vi "Controller.vi"(8 "error in":errorcluster) -> ()   [LabVIEW 2014, in "Elevator System.lvlib"]
uses:
  Elevator System.lvlib
  Typedef/MessageType.ctl
  Typedef/Commands.ctl
  Typedef/GripperNotifierType.ctl
  Typedef/ControllerStateData.ctl
  Typedef/ControllerStates.ctl
  Typedef/StackMessage.ctl
  Typedef/StackCommandType.ctl
  Typedef/TeirNumber.ctl
  Sensors Global.vi
panel:
  in  "Loops":i32=7
  in  "Tolerance 2":dbl=0.015 format="%#_13g"
  in  "Tolerance":dbl=0.04 format="%#_13g"
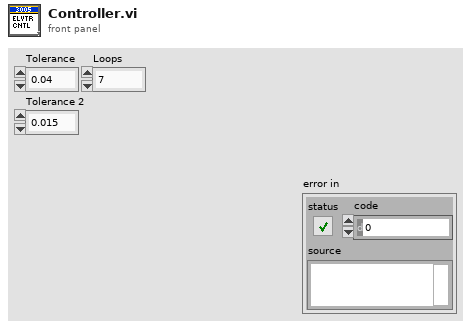
[diagram p1: front panel]
types:
  T1 = typedef "Elevator System.lvlib/ControllerStates.ctl" = enum16{"Init", "Set Elevator SP", "Set Gripper SP", "Wait For Elevator", "Wait For Gripper", "Wait For Elevator Fast", "Wait For Gripper Fast", "Disabled"}
  T2 = typedef "Elevator System.lvlib/ControllerStateData.ctl" = cluster{"State":T1, "Data":dbl[]}
  T3 = cluster{"Elevator":refnum<notifier>, "Gripper":refnum<notifier>}
  T4 = typedef "Elevator System.lvlib/Commands.ctl" = enum16{"Home", "Stack", "Pickup", "Score", "Cycle", "Stop", "Manual Open", "Manual Close", "Manual Up", "Manual Down", "Gripper RC", "Gripper Cycle", "Wait On Gripper", "Wait On Elevator"}
  T5 = typedef "Elevator System.lvlib/MessageType.ctl" = cluster{"Name":T4, "Data":variant}
  T6 = typedef "Elevator System.lvlib/StackMessage.ctl" = cluster{"Type":T7, "Teir":T8}
  T7 = typedef "Elevator System.lvlib/StackCommandType.ctl" = enum16{"Normal", "RC", "Step"}
  T8 = typedef "Elevator System.lvlib/TeirNumber.ctl" = enum16{"T1", "T2", "T3", "T4", "T5", "T6"}
  T9 = typedef "Elevator System.lvlib/GripperNotifierType.ctl" = cluster{"SP Left":dbl, "SP Right":dbl}
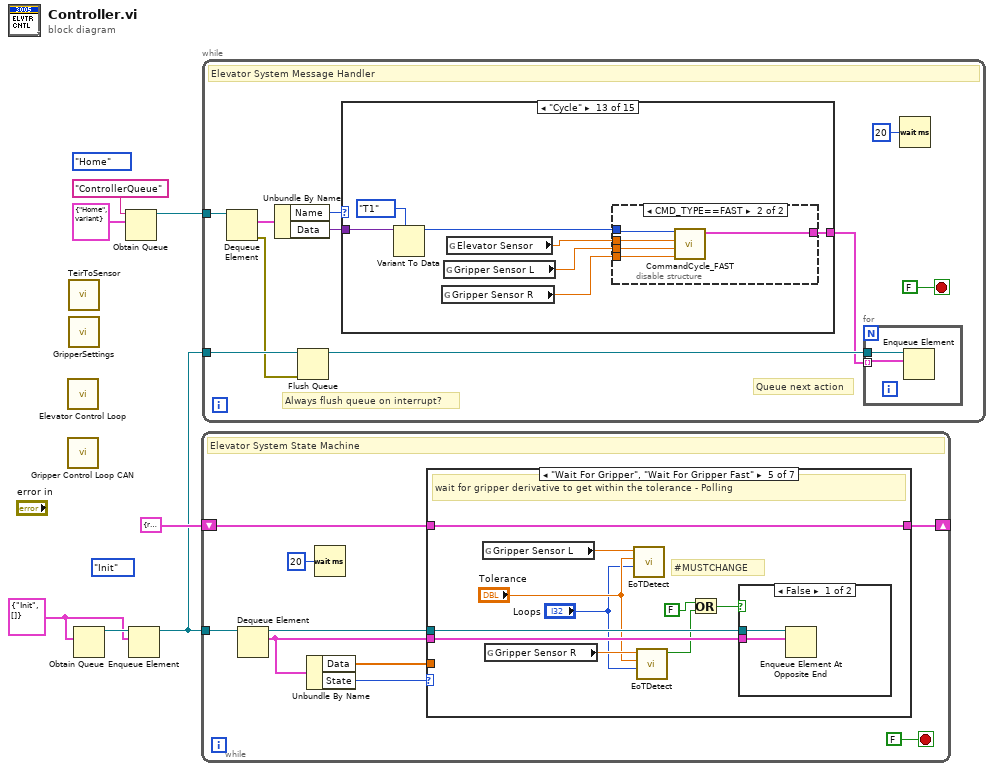
[diagram p0: block diagram]
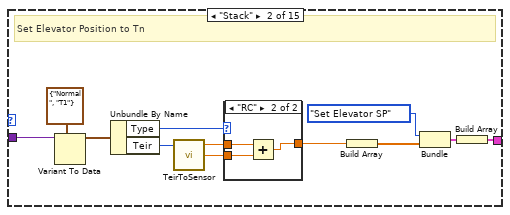
[diagram p3: hidden frame]
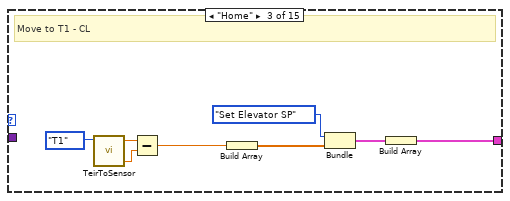
[diagram p5: hidden frame]
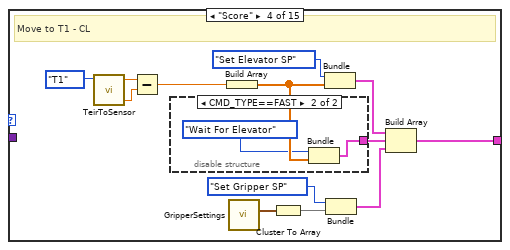
[diagram p6: hidden frame]
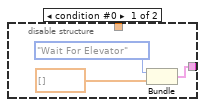
[diagram p7: hidden frame]
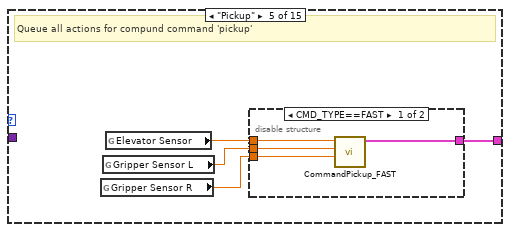
[diagram p8: hidden frame]
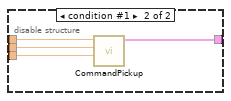
[diagram p9: hidden frame]
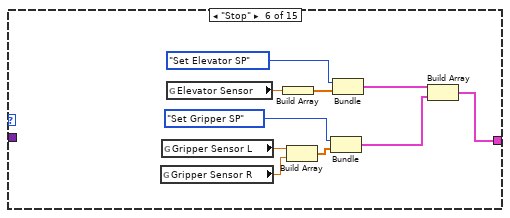
[diagram p10: hidden frame]
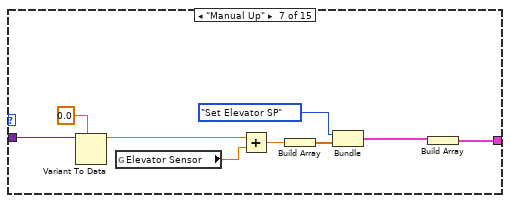
[diagram p11: hidden frame]
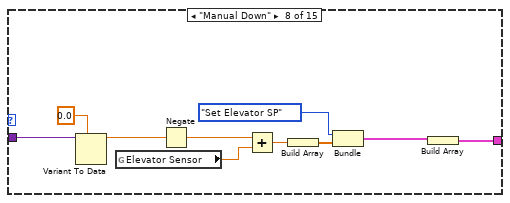
[diagram p12: hidden frame]
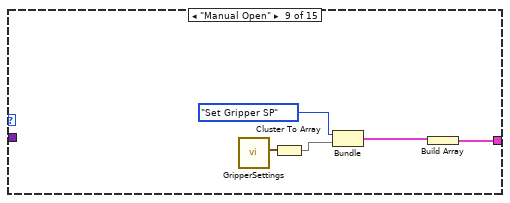
[diagram p13: hidden frame]
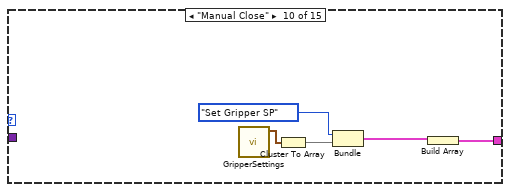
[diagram p14: hidden frame]
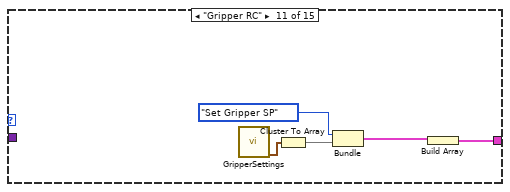
[diagram p15: hidden frame]
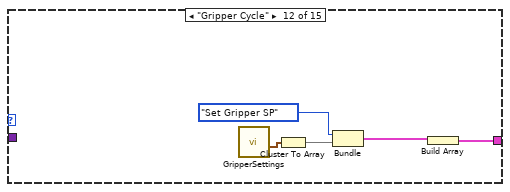
[diagram p16: hidden frame]
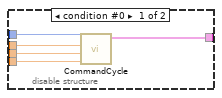
[diagram p17: hidden frame]
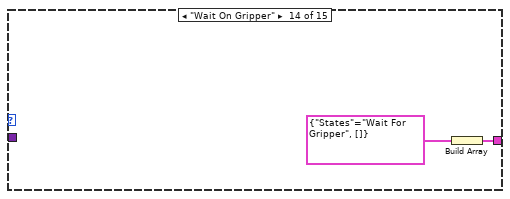
[diagram p18: hidden frame]
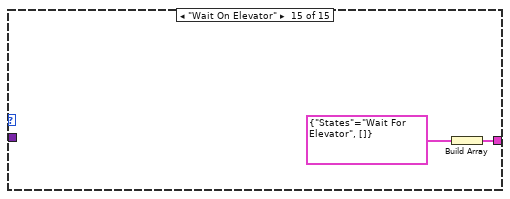
[diagram p19: hidden frame]
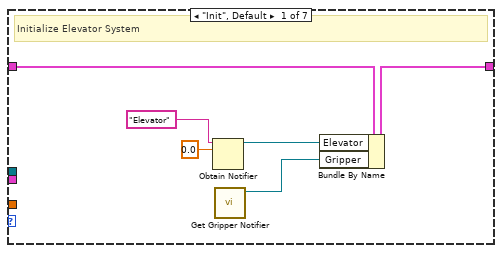
[diagram p20: hidden frame]
diagram:
  (unwired) ControllerStates."Init" ("State")
  w1 = T2 {"State"=enum."Init", "Data"=[]}
  (unwired) Commands."Home" ("Name")
  n1 = call "Elevator Control Loop.vi"() -> ()  [unwired: 12 in]
  n2 = call "Gripper Control Loop CAN.vi"() -> ()  [unwired: 12 in]
  n3 = call "TeirToSensor.vi"() -> ()  [unwired: 4 in, 5 out]
  n4 = call "GripperSettings.vi"() -> ()  [unwired: 5 in, 5 out]
  n5 = Obtain Queue(element data type=w1) -> (queue out=w4:refnum<queue>)  [unwired: 4 in, 2 out]
  n6 = Obtain Queue(name (unnamed)="ControllerQueue", element data type=T5 {"Name"=enum."Home", "Data"=variant} ("Message")) -> (queue out=w5:refnum<queue>)  [unwired: 3 in, 2 out]
  n7 = Enqueue Element(queue=w4, element=w1) -> (queue out=w2:refnum<queue>)  [unwired: 2 in, 2 out]
  n8 = while {
    tunnel: w2 -> [w14]
    shift-right: [w11] -> _
    shift-left: T3 {"Elevator"=refnum, "Gripper"=refnum} -> [w12]
    stop <- FALSE stop-if-true
    # "Elevator System State Machine"
    n9 = Dequeue Element(queue=w14) -> (queue out=w13:refnum<queue>, element=w10:T2)  [unwired: 2 in, 2 out]
    n10 = Unbundle By Name(w10) -> ("Data"=w8:dbl[], "State"=w9:T1)
    n11 = Wait (ms)(milliseconds to wait=u32 20) -> ()  [unwired: 1 out]
    n12 = case shown="\"Wait For Gripper\", \"Wait For Gripper Fast\"" w9 {
      tunnel: w13 -> [_ _ _ w36 w50 w65 w86]
      tunnel: w12 -> [w20 w29 w33 w39 w52 w66 w87]
      tunnel: [w19 w29 w33 w39 w52 w66 w87] -> w11
      tunnel: w10 -> [_ _ _ w35 w49 w64 w85]
      tunnel: w8 -> [_ w24 w30 _ _ w63 w77]
      frame "Init", Default {
        # "Initialize Elevator System"
        n13 = Obtain Notifier(name (unnamed)="Elevator", notification data type=0.0) -> (notifier out=w21:refnum<notifier>)  [unwired: 2 in, 2 out]
        n14 = call "Get Gripper Notifier.vi"() -> ("Notifier out"=w17:refnum<notifier>)  [unwired: 11 in]
        n15 = Bundle By Name(cluster=w20, "Elevator"=w21, "Gripper"=w17) -> (w19:T3)
      }
      frame "Set Elevator SP" {
        # "Set the Elevator PID Setpoint"
        n16 = Index Array(array=w24) -> (element=w23:dbl)  [unwired: 1 in]
        n17 = call "TeirToSensor.vi"() -> ("Max"=w26:dbl, "Min"=w25:dbl)  [unwired: 4 in, 3 out]
        n18 = Unbundle By Name(w29) -> ("Elevator"=w28:refnum<notifier>)
        n19 = In Range and Coerce(upper limit=w26, x=w23, lower limit=w25) -> (coerced(x)=w27:dbl)  [unwired: 1 out]
        n20 = Send Notification(notification=w27, notifier=w28) -> ()  [unwired: 1 in, 2 out]
      }
      frame "Set Gripper SP" {
        # "Set the Gripper PID Setpoint"
        n21 = Array To Cluster(array=w30) -> (cluster=w31:cluster{"Data[0]":dbl, "Data[1]":dbl})
        n22 = Unbundle By Name(w33) -> ("Gripper"=w32:refnum<notifier>)
        n23 = Send Notification(notification=w31, notifier=w32) -> ()  [unwired: 1 in, 2 out]
      }
      frame "Wait For Elevator" {
        # "wait for elevator derivative to get within the tolerance - Polling"
        n24 = global read "Sensors Global.vi" "Elevator Sensor"() -> (w38:dbl)
        n25 = call "EoTDetect.vi"("Tolerance"="Tolerance 2", "Sensor"=w38) -> ("EoT? (F)"=w34:bool)  [unwired: 9 in]
        n26 = case shown="False" w34 {
          tunnel: w36 -> [w41 _]
          tunnel: w35 -> [w40 _]
          frame False {
            n27 = Enqueue Element At Opposite End(queue=w41, element=w40) -> ()  [unwired: 2 in, 3 out]
          }
          frame True {
            n28 = call "GetElevatorStatus.vi"("Action"=enum16{"Get", "Set", "Clear"}."Set") -> ()  [unwired: 10 in, 1 out]
          }
        }
      }
      frame "Wait For Gripper", "Wait For Gripper Fast" {
        # "#MUSTCHANGE"
        # "wait for gripper derivative to get within the tolerance - Polling"
        n29 = global read "Sensors Global.vi" "Gripper Sensor L"() -> (w51:dbl)
        n30 = global read "Sensors Global.vi" "Gripper Sensor R"() -> (w48:dbl)
        n31 = call "EoTDetect.vi"("Loops"="Loops", "Tolerance"="Tolerance", "Sensor"=w51) -> ()  [unwired: 8 in, 1 out]
        n32 = call "EoTDetect.vi"("Loops"="Loops", "Tolerance"="Tolerance", "Sensor"=w48) -> ("EoT? (F)"=w44:bool)  [unwired: 8 in]
        n33 = Or(x=FALSE ("y"), y=w44) -> (x .or. y?=w47:bool)
        n34 = case shown="False" w47 {
          tunnel: w50 -> [w54 _]
          tunnel: w49 -> [w53 _]
          frame False {
            n35 = Enqueue Element At Opposite End(queue=w54, element=w53) -> ()  [unwired: 2 in, 3 out]
          }
          frame True {
            n36 = call "GetGripperStatus.vi"("Action"=enum16{"Get", "Set", "Clear"}."Set") -> ()  [unwired: 10 in, 1 out]
          }
        }
      }
      frame "Wait For Elevator Fast" {
        # "-1 = Going Down\n1 = going up"
        # "Wait for Elevator to get to a position - Polling"
        n37 = call "TeirToSensor.vi"() -> ("Max"=w58:dbl)  [unwired: 4 in, 4 out]
        n38 = global read "Sensors Global.vi" "Elevator Sensor"() -> (w62:dbl)
        n39 = Index Array(array=w63) -> (element #1=w61:dbl, element #2=w56:dbl)  [unwired: 2 in]
        n40 = In Range and Coerce(upper limit=w58, x=w61, lower limit=0.3) -> (coerced(x)=w59:dbl)  [unwired: 1 out]
        n41 = case shown="-1, Default" w56 {
          tunnel: w62 -> [w69 w72]
          tunnel: w59 -> [w68 w71]
          tunnel: [w67 w70] -> w60
          frame 1 {
            n42 = Greater Or Equal?(x=w69, y=w68) -> (x >= y?=w67:bool)
          }
          frame -1, Default {
            n43 = Less Or Equal?(x=w72, y=w71) -> (x <= y?=w70:bool)
          }
        }
        n44 = case shown="False" w60 {
          tunnel: w65 -> [w74 _]
          tunnel: w64 -> [w73 _]
          frame False {
            n45 = Enqueue Element At Opposite End(queue=w74, element=w73) -> ()  [unwired: 2 in, 3 out]
          }
          frame True {
            n46 = call "GetElevatorStatus.vi"("Action"=enum16{"Get", "Set", "Clear"}."Set") -> ()  [unwired: 10 in, 1 out]
          }
        }
      }
      frame "Disabled" {
        # "Wait for Elevator to get to target position - Polling"
        n47 = global read "Sensors Global.vi" "Gripper Sensor L"() -> (w82:dbl)
        n48 = global read "Sensors Global.vi" "Gripper Sensor R"() -> (w81:dbl)
        n49 = Build Array(w82, w81) -> (w80:dbl[])
        n50 = Subtract(x=w80, y=w77) -> (x-y=w84:dbl[])
        n51 = Absolute Value(x=w84) -> (abs(x)=w83:dbl[])
        n52 = call "GripperSettings.vi"() -> ("Detect Tolerance"=w76:dbl)  [unwired: 5 in, 4 out]
        n53 = Less?(x=w83, y=w76) -> (x < y?=w78:bool[])
        n54 = And Array Elements(Boolean array=w78) -> (logical AND=w79:bool)
        n55 = case shown="False" w79 {
          tunnel: w86 -> [w89 _]
          tunnel: w85 -> [w88 _]
          frame False {
            n56 = Enqueue Element At Opposite End(queue=w89, element=w88) -> ()  [unwired: 2 in, 3 out]
          }
          frame True {
            n57 = call "GetElevatorStatus.vi"("Action"=enum16{"Get", "Set", "Clear"}."Set") -> ()  [unwired: 10 in, 1 out]
          }
        }
      }
    }
  }
  n58 = while {
    tunnel: w5 -> [w96]
    tunnel: w2 -> [w97]
    stop <- FALSE stop-if-true
    # "Queue next action"
    # "Always flush queue on interrupt?"
    # "Elevator System Message Handler"
    n59 = Dequeue Element(queue=w96) -> (element=w95:T5, error out=w92:errorcluster)  [unwired: 2 in, 2 out]
    n60 = Unbundle By Name(w95) -> ("Name"=w99:T4, "Data"=w98:variant)
    n61 = Flush Queue(queue=w97, error in (no error)=w92) -> (queue out=w100:refnum<queue>)  [unwired: 2 out]
    n62 = case shown="\"Cycle\"" w99 {
      tunnel: w98 -> [_ w112 _ _ _ _ w169 w179 _ _ _ _ w208 _ _]
      tunnel: [_ w109 w122 w135 w147 w163 w172 w182 w187 w192 w197 w202 w211 w222 w224] -> w94
      frame Default {
      }
      frame "Stack" {
        # "Set Elevator Position to Tn"
        n63 = Variant To Data(type=T6 {"Type"=enum."Normal", "Teir"=enum."T1"}, Variant=w112) -> (data=w107:T6)  [unwired: 1 in, 1 out]
        n64 = Unbundle By Name(w107) -> ("Type"=w102:T7, "Teir"=w106:T8)
        n65 = call "TeirToSensor.vi"("Enum"=w106) -> ("T1"=w105:dbl, "CR"=w104:dbl)  [unwired: 3 in, 3 out]
        n66 = case shown="\"RC\"" w102 {
          tunnel: w105 -> [w113 w116]
          tunnel: w104 -> [_ w115]
          tunnel: [w113 w114] -> w103
          frame "Normal", Default {
          }
          frame "RC" {
            n67 = Add(x=w116, y=w115) -> (x+y=w114:dbl)
          }
        }
        n68 = Build Array(w103) -> (w101:dbl[])
        n69 = Bundle("States"=ControllerStates."Set Elevator SP", w101) -> (w110:cluster{"States":T1, dbl[]})  [unwired: 1 in]
        n70 = Build Array(w110) -> (w109:cluster{"States":T1, dbl[]}[])
      }
      frame "Home" {
        # "Move to T1 - CL"
        n71 = call "TeirToSensor.vi"("Enum"=TeirNumber."T1") -> ("T1"=w120:dbl, "CL"=w119:dbl)  [unwired: 3 in, 3 out]
        n72 = Subtract(x=w120, y=w119) -> (x-y=w118:dbl)
        n73 = Build Array(w118) -> (w117:dbl[])
        n74 = Bundle("States"=ControllerStates."Set Elevator SP", w117) -> (w123:cluster{"States":T1, dbl[]})  [unwired: 1 in]
        n75 = Build Array(w123) -> (w122:cluster{"States":T1, dbl[]}[])
      }
      frame "Score" {
        # "Move to T1 - CL"
        n76 = call "TeirToSensor.vi"("Enum"=TeirNumber."T1") -> ("T1"=w133:dbl, "CL"=w132:dbl)  [unwired: 3 in, 3 out]
        n77 = Subtract(x=w133, y=w132) -> (x-y=w129:dbl)
        n78 = Build Array(w129) -> (w125:dbl[])
        n79 = disable-structure shown="CMD_TYPE==FAST" {
          disable-tunnel: [w139 w143] -> w128
          disable-tunnel: w125 -> [_ w142]
          frame condition #0 {
            n80 = Bundle("States"=ControllerStates."Wait For Elevator", dbl[] []) -> (w139:cluster{"States":T1, dbl[]})  [unwired: 1 in]
          }
          frame condition #1 (active) {
            n81 = Bundle("States"=ControllerStates."Wait For Elevator", w142) -> (w143:cluster{"States":T1, dbl[]})  [unwired: 1 in]
          }
        }
        n82 = call "GripperSettings.vi"() -> ("Open"=w127:T9)  [unwired: 5 in, 4 out]
        n83 = Cluster To Array(cluster=w127) -> (array=w126:dbl[])
        n84 = Bundle("States"=ControllerStates."Set Elevator SP", w125) -> (w136:cluster{"States":T1, dbl[]})  [unwired: 1 in]
        n85 = Bundle("States"=ControllerStates."Set Gripper SP", "Open"=w126) -> (w130:cluster{"States":T1, "Open":dbl[]})  [unwired: 1 in]
        n86 = Build Array(w136, w128, w130) -> (w135:cluster{"States":T1, "Open":dbl[]}[])
      }
      frame "Pickup" {
        # "Queue all actions for compund command 'pickup'"
        n87 = global read "Sensors Global.vi" "Gripper Sensor R"() -> (w144:dbl)
        n88 = global read "Sensors Global.vi" "Gripper Sensor L"() -> (w145:dbl)
        n89 = global read "Sensors Global.vi" "Elevator Sensor"() -> (w146:dbl)
        n90 = disable-structure shown="CMD_TYPE==FAST" {
          disable-tunnel: [w148 w155] -> w147
          disable-tunnel: w146 -> [w151 w154]
          disable-tunnel: w145 -> [w149 w153]
          disable-tunnel: w144 -> [w150 w152]
          frame condition #0 (active) {
            n91 = call "CommandPickup_FAST.vi"("Gripper Value R"=w150, "Gripper Value L"=w149, "Elevator Value"=w151) -> ("appended array"=w148:cluster{"States":T1, "Close":dbl[]}[])  [unwired: 8 in]
          }
          frame condition #1 {
            n92 = call "CommandPickup.vi"("Gripper Value R"=w152, "Gripper Value L"=w153, "Elevator Value"=w154) -> ("appended array"=w155:cluster{"States":T1, "Close":dbl[]}[])  [unwired: 8 in]
          }
        }
      }
      frame "Stop" {
        n93 = global read "Sensors Global.vi" "Gripper Sensor R"() -> (w157:dbl)
        n94 = global read "Sensors Global.vi" "Gripper Sensor L"() -> (w158:dbl)
        n95 = global read "Sensors Global.vi" "Elevator Sensor"() -> (w162:dbl)
        n96 = Build Array(w162) -> (w159:dbl[])
        n97 = Build Array(w158, w157) -> (w156:dbl[])
        n98 = Bundle("States"=ControllerStates."Set Gripper SP", w156) -> (w160:cluster{"States":T1, dbl[]})  [unwired: 1 in]
        n99 = Bundle("States"=ControllerStates."Set Elevator SP", w159) -> (w164:cluster{"States":T1, dbl[]})  [unwired: 1 in]
        n100 = Build Array(w164, w160) -> (w163:cluster{"States":T1, dbl[]}[])
      }
      frame "Manual Up" {
        n101 = Variant To Data(type=0.0, Variant=w169) -> (data=w167:dbl)  [unwired: 1 in, 1 out]
        n102 = global read "Sensors Global.vi" "Elevator Sensor"() -> (w171:dbl)
        n103 = Add(x=w167, y=w171) -> (x+y=w170:dbl)
        n104 = Build Array(w170) -> (w166:dbl[])
        n105 = Bundle("States"=ControllerStates."Set Elevator SP", w166) -> (w173:cluster{"States":T1, dbl[]})  [unwired: 1 in]
        n106 = Build Array(w173) -> (w172:cluster{"States":T1, dbl[]}[])
      }
      frame "Manual Down" {
        n107 = Variant To Data(type=0.0, Variant=w179) -> (data=w177:dbl)  [unwired: 1 in, 1 out]
        n108 = global read "Sensors Global.vi" "Elevator Sensor"() -> (w181:dbl)
        n109 = Negate(x=w177) -> (-x=w176:dbl)
        n110 = Add(x=w176, y=w181) -> (x+y=w180:dbl)
        n111 = Build Array(w180) -> (w175:dbl[])
        n112 = Bundle("States"=ControllerStates."Set Elevator SP", w175) -> (w183:cluster{"States":T1, dbl[]})  [unwired: 1 in]
        n113 = Build Array(w183) -> (w182:cluster{"States":T1, dbl[]}[])
      }
      frame "Manual Open" {
        n114 = call "GripperSettings.vi"() -> ("Open"=w186:T9)  [unwired: 5 in, 4 out]
        n115 = Cluster To Array(cluster=w186) -> (array=w185:dbl[])
        n116 = Bundle("States"=ControllerStates."Set Gripper SP", "Open"=w185) -> (w188:cluster{"States":T1, "Open":dbl[]})  [unwired: 1 in]
        n117 = Build Array(w188) -> (w187:cluster{"States":T1, "Open":dbl[]}[])
      }
      frame "Manual Close" {
        n118 = call "GripperSettings.vi"() -> ("Close"=w191:T9)  [unwired: 5 in, 4 out]
        n119 = Cluster To Array(cluster=w191) -> (array=w190:dbl[])
        n120 = Bundle("States"=ControllerStates."Set Gripper SP", "Close"=w190) -> (w193:cluster{"States":T1, "Close":dbl[]})  [unwired: 1 in]
        n121 = Build Array(w193) -> (w192:cluster{"States":T1, "Close":dbl[]}[])
      }
      frame "Gripper RC" {
        n122 = call "GripperSettings.vi"() -> ("RC"=w195:T9)  [unwired: 5 in, 4 out]
        n123 = Cluster To Array(cluster=w195) -> (array=w196:dbl[])
        n124 = Bundle("States"=ControllerStates."Set Gripper SP", "RC"=w196) -> (w198:cluster{"States":T1, "RC":dbl[]})  [unwired: 1 in]
        n125 = Build Array(w198) -> (w197:cluster{"States":T1, "RC":dbl[]}[])
      }
      frame "Gripper Cycle" {
        n126 = call "GripperSettings.vi"() -> ("Cycle"=w200:T9)  [unwired: 5 in, 4 out]
        n127 = Cluster To Array(cluster=w200) -> (array=w201:dbl[])
        n128 = Bundle("States"=ControllerStates."Set Gripper SP", "Cycle"=w201) -> (w203:cluster{"States":T1, "Cycle":dbl[]})  [unwired: 1 in]
        n129 = Build Array(w203) -> (w202:cluster{"States":T1, "Cycle":dbl[]}[])
      }
      frame "Cycle" {
        n130 = Variant To Data(type=TeirNumber."T1" ("data"), Variant=w208) -> (data=w206:T8)  [unwired: 1 in, 1 out]
        n131 = global read "Sensors Global.vi" "Gripper Sensor R"() -> (w205:dbl)
        n132 = global read "Sensors Global.vi" "Gripper Sensor L"() -> (w210:dbl)
        n133 = global read "Sensors Global.vi" "Elevator Sensor"() -> (w209:dbl)
        n134 = disable-structure shown="CMD_TYPE==FAST" {
          disable-tunnel: [w216 w220] -> w211
          disable-tunnel: w210 -> [w215 w218]
          disable-tunnel: w209 -> [w214 w219]
          disable-tunnel: w206 -> [w213 w221]
          disable-tunnel: w205 -> [w212 w217]
          frame condition #0 {
            n135 = call "CommandCycle.vi"("Gripper Value R"=w212, "Gripper Value L"=w215, "Elevator Value"=w214, "Teir Selection"=w213) -> ("appended array"=w216:cluster{"States":T1, "Close":dbl[]}[])  [unwired: 7 in]
          }
          frame condition #1 (active) {
            n136 = call "CommandCycle_FAST.vi"("Gripper Value R"=w217, "Gripper Value L"=w218, "Elevator Value"=w219, "Teir Selection"=w221) -> ("appended array"=w220:cluster{"States":T1, "Close":dbl[]}[])  [unwired: 7 in]
          }
        }
      }
      frame "Wait On Gripper" {
        n137 = Build Array(cluster{"States":T1, dbl[]} {"States"=enum."Wait For Gripper", []}) -> (w222:cluster{"States":T1, dbl[]}[])
      }
      frame "Wait On Elevator" {
        n138 = Build Array(cluster{"States":T1, dbl[]} {"States"=enum."Wait For Elevator", []}) -> (w224:cluster{"States":T1, dbl[]}[])
      }
    }
    n139 = for {
      tunnel: w100 -> [w227]
      tunnel: w94 -> [w226] mode=indexing
      n140 = Enqueue Element(queue=w227, element=w226) -> ()  [unwired: 2 in, 3 out]
    }
    n141 = Wait (ms)(milliseconds to wait=u32 20) -> ()  [unwired: 1 out]
  }
